vi "Filter SwitchActionList.vi"(7 "Relay Counts":i32[](array[numeric]), 8 "error in (no error)":errorcluster, 9 "Relay Indexes":i32[](array[numeric]), 10 "SwitchActionList in":T1[](array[typedef]) {"relay action" items=["CloseRelay"=21, "OpenRelay"=20]}, 11 "SLSC Switch in":refnum<class "SLSC Switch.lvclass">) -> (0 "error out":errorcluster, 2 "SwitchActionList out":T1[](array[typedef]) {"relay action" items=["CloseRelay"=21, "OpenRelay"=20]}, 3 "SLSC Switch out":refnum<class "SLSC Switch.lvclass">)   [LabVIEW 2016, in "SLSC Switch.lvlib" / "SLSC Switch.lvclass"]
uses:
  SLSC Switch.lvclass
  Switch Action Processor/controls/Switch Action.ctl
  Relay/Relay Action.ctl
  Relay/Relay.lvclass
  Switch Action Processor/Switch Action Processor.lvclass
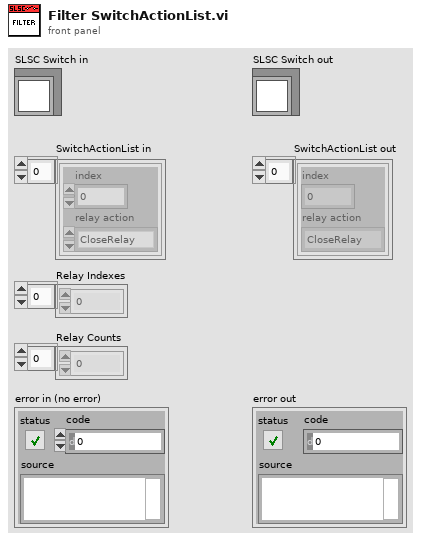
[diagram p1: front panel]
types:
  T1 = typedef "SLSC Switch.lvlib/Switch Action Processor.lvclass/Switch Action.ctl" = cluster{"index":i32, "relay action":T2}
  T2 = typedef "SLSC Switch.lvlib/Relay.lvclass/Relay Action.ctl" = u32
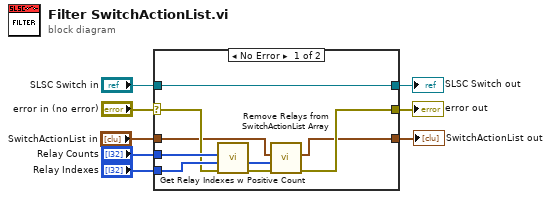
[diagram p0: block diagram]
diagram:
  n1 = case shown="No Error" "error in (no error)" {
    selector: "error in (no error)" -> [w13 w20]
    tunnel: "Relay Indexes" -> [w15 _]
    tunnel: [w12 w20] -> w7
    tunnel: [w9 w19] -> w1
    tunnel: "SwitchActionList in" -> [w10 w19]
    tunnel: "SLSC Switch in" -> [w11 w18]
    tunnel: [w11 w18] -> w4
    tunnel: "Relay Counts" -> [w14 _]
    frame No Error {
      n2 = call "Get Relay Indexes w Positive Count.vi"("error in (no error)"=w13, "Relay Indexes"=w15, "Relay Counts"=w14) -> ("error out"=w17:errorcluster, "Positive Relay Count Array"=w16:i32[])  [unwired: 7 in]
      n3 = call "Remove Relays from SwitchActionList Array.vi"("error in (no error)"=w17, "Relay Count Subarray [Count>0]"=w16, "SwitchActionList in"=w10) -> ("error out"=w12:errorcluster, "SwitchActionList out"=w9:T1[])  [unwired: 6 in, 1 out]
    }
    frame Error {
    }
  }
  "error out" <- w7
  "SLSC Switch out" <- w4
  "SwitchActionList out" <- w1
